vi "get source name.vi"(8 "error in":errorcluster, 11 "timing source in":refnum<class "usec timing source.lvclass">) -> (0 "error out":errorcluster, 2 "source name":string, 3 "timing source out":refnum<class "usec timing source.lvclass">)   [LabVIEW 2013, in "usec timing source.lvclass"]
doc: "Returns the name of the timing source to be used as part of the configuration of a timed loop. For example, the 1 ms timer would return the string \"1 kHz\"."
uses:
  usec timing source.lvclass
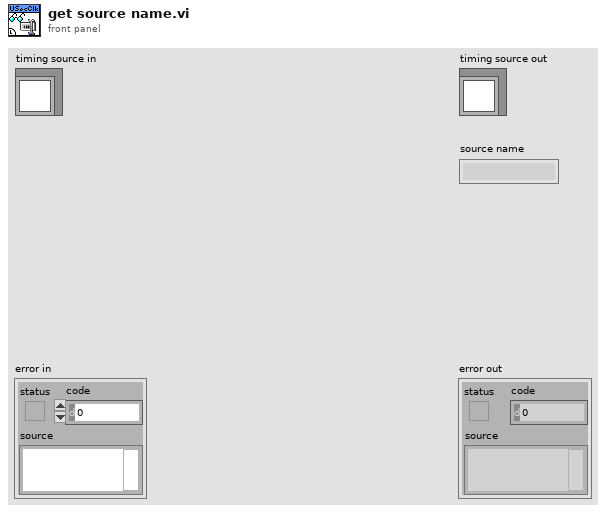
[diagram p1: front panel]
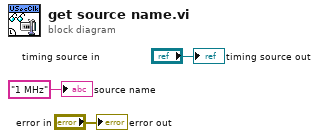
[diagram p0: block diagram]
diagram:
  "error out" <- "error in"
  "timing source out" <- "timing source in"
  "source name" <- "1 MHz" ("source name")
